vi "initalize dual gating(SubVI).vi"(0 "簇":T1={"initialize"=enum."SR830", "6221"={"6221 Resource"="GPIB0::24::INSTR", "Delta status"=FALSE, "电流"=0.0}, "SR830+6221"={"source"=0, "阻抗"=0.0, "量程入 4"=0, "量程入 3"=0, "量程入 2"=0, "量程入 1"=0, "SR830 2"=FALSE, "SR830 3"=FALSE, "SR830 4"=FALSE, "SR830 1"=FALSE, "VISA 1"="", "VISA 2"="", "VISA 3"="", "VISA 4"="", "Reserve 1"=0, "Reserve 2"=-1, "Reserve 3"=-1, "Reserve 4"=-1, "量程"=enum."量程每次测量会判定"}, "2400"={"2400"=FALSE, "VISA"=""}, "ch"={"ch"=[], "current"=[], "change?"=[], "holding current\nwhen change ch?"=FALSE}, "Instrument"={"335 Resource"="GPIB0::24::INSTR", "Input (0:A)"=0, "Instrument Type"=enum."SVSM", "quantum design"=refnum, "Heater Output (1:1)"=1, "semaphore"=refnum, "TCP master instance"=refnum, "335 Status"=refnum, "M24C Resource"="GPIB0::24::INSTR", "4G supply"="GPIB0::24::INSTR", "Temp Status 24C"=refnum, "Temp"=refnum, "9T信号"=refnum, "limit"={"Field limit"=0.0, "Field rate limit"=0.0, "Temp limit"=0.0, "Temp low limit"=0.0, "Temp rate limit "=0.0}, "4g supply status"=refnum, "vi路径"=""}, "Aborting"=refnum, "数据文件"=refnum, "warning"=refnum, "2614B"={"2614B chA"=FALSE, "2614B chB"=FALSE, "VISA"=""}} {"Instrument"."Input (0:A)" items=["A", "B"]; "Instrument"."Heater Output (1:1)" items=["1"=1, "2"=2]; "SR830+6221"."Reserve 4" items=["Auto Reserve"=-1, "High Reserve"=0, "Normal"=1, "Low Noise"=2]; "SR830+6221"."Reserve 3" items=["Auto Reserve"=-1, "High Reserve"=0, "Normal"=1, "Low Noise"=2]; "SR830+6221"."Reserve 2" items=["Auto Reserve"=-1, "High Reserve"=0, "Normal"=1, "Low Noise"=2]; "SR830+6221"."Reserve 1" items=["量程每次测量会判定", "量程不变为设定值"]; "SR830+6221"."source" items=["SR830 1", "SR830 2", "SR830 3", "SR830 4"]}, 2 "字符串":string) -> (7 "输出簇":T1={"initialize"=enum."SR830", "6221"={"6221 Resource"="GPIB0::24::INSTR", "Delta status"=FALSE, "电流"=0.0}, "SR830+6221"={"source"=0, "阻抗"=0.0, "量程入 4"=0, "量程入 3"=0, "量程入 2"=0, "量程入 1"=0, "SR830 2"=FALSE, "SR830 3"=FALSE, "SR830 4"=FALSE, "SR830 1"=FALSE, "VISA 1"="", "VISA 2"="", "VISA 3"="", "VISA 4"="", "Reserve 1"=0, "Reserve 2"=-1, "Reserve 3"=-1, "Reserve 4"=-1, "量程"=enum."量程每次测量会判定"}, "2400"={"2400"=FALSE, "VISA"=""}, "ch"={"ch"=[], "current"=[], "change?"=[], "holding current\nwhen change ch?"=FALSE}, "Instrument"={"335 Resource"="GPIB0::24::INSTR", "Input (0:A)"=0, "Instrument Type"=enum."SVSM", "quantum design"=refnum, "Heater Output (1:1)"=1, "semaphore"=refnum, "TCP master instance"=refnum, "335 Status"=refnum, "M24C Resource"="GPIB0::24::INSTR", "4G supply"="GPIB0::24::INSTR", "Temp Status 24C"=refnum, "Temp"=refnum, "9T信号"=refnum, "limit"={"Field limit"=0.0, "Field rate limit"=0.0, "Temp limit"=0.0, "Temp low limit"=0.0, "Temp rate limit "=0.0}, "4g supply status"=refnum, "vi路径"=""}, "Aborting"=refnum, "数据文件"=refnum, "warning"=refnum, "2614B"={"2614B chA"=FALSE, "2614B chB"=FALSE, "VISA"=""}} {"Instrument"."Input (0:A)" items=["A", "B"]; "Instrument"."Heater Output (1:1)" items=["1"=1, "2"=2]; "SR830+6221"."Reserve 4" items=["Auto Reserve"=-1, "High Reserve"=0, "Normal"=1, "Low Noise"=2]; "SR830+6221"."Reserve 3" items=["Auto Reserve"=-1, "High Reserve"=0, "Normal"=1, "Low Noise"=2]; "SR830+6221"."Reserve 2" items=["Auto Reserve"=-1, "High Reserve"=0, "Normal"=1, "Low Noise"=2]; "SR830+6221"."Reserve 1" items=["量程每次测量会判定", "量程不变为设定值"]; "SR830+6221"."source" items=["SR830 1", "SR830 2", "SR830 3", "SR830 4"]})   [LabVIEW 2019, in "initialize.lvlib"]
uses:
  initialize.lvlib
  config.ctl
  <vilib>/NI/Modbus Library/API/Master/Modbus Master.lvclass
  initialize.ctl
  Instrument.ctl
  Instrument Type.ctl
  lib/QDInstrument.dll
  335 state.ctl
  limit.ctl
  9T mag field stauts.ctl
  warning.ctl
  lib/Keithley 2600 Series/Public/Configure/Source/Configure Source (Range).vi
  lib/Keithley 2600 Series/Public/Configure/Source/Configure Source (Limit).vi
  lib/Keithley 2600 Series/Keithley 2600 Series.lvlib
panel:
  in  "chB":bool
  in  "chA":bool
  in  "Current Limit B (0.1 A) 2":dbl=0.1
  in  "Current Limit A (0.1 A)":dbl=0.1
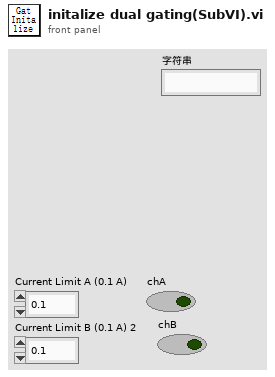
[diagram p1: front panel]
types:
  T1 = typedef "config.ctl" = cluster{"initialize":T2, "6221":cluster{"6221 Resource":refnum<visa-resource-name>, "Delta status":bool, "电流":dbl}, "SR830+6221":cluster{"source":u16, "阻抗":dbl, "量程入 4":i32, "量程入 3":i32, "量程入 2":i32, "量程入 1":i32, "SR830 2":bool, "SR830 3":bool, "SR830 4":bool, "SR830 1":bool, "VISA 1":refnum<visa-resource-name>, "VISA 2":refnum<visa-resource-name>, "VISA 3":refnum<visa-resource-name>, "VISA 4":refnum<visa-resource-name>, "Reserve 1":i16, "Reserve 2":i16, "Reserve 3":i16, "Reserve 4":i16, "量程":enum16{"量程每次测量会判定", "量程不变为设定值"}}, "2400":cluster{"2400":bool, "VISA":refnum<visa-resource-name>}, "ch":cluster{"ch":i32[], "current":dbl[], "change?":bool[], "holding current\nwhen change ch?":bool}, "Instrument":T3, "Aborting":refnum<vi>, "数据文件":refnum<vi>, "warning":refnum<vi>, "2614B":cluster{"2614B chA":bool, "2614B chB":bool, "VISA":refnum<visa-resource-name>}}
  T2 = typedef "initialize.ctl" = enum16{"SR830", "keithley6221-SR830", "Delta", "Delta-tunnelling", "keithley6221-2182-DC"}
  T3 = typedef "Instrument.ctl" = cluster{"335 Resource":refnum<visa-resource-name>, "Input (0:A)":u16, "Instrument Type":T4, "quantum design":refnum<k24>, "Heater Output (1:1)":u16, "semaphore":T5, "TCP master instance":refnum<class "Modbus Master.lvclass">, "335 Status":refnum<vi>, "M24C Resource":refnum<visa-resource-name>, "4G supply":refnum<visa-resource-name>, "Temp Status 24C":refnum<vi>, "Temp":refnum<vi>, "9T信号":T5, "limit":T6, "4g supply status":refnum<vi>, "vi路径":string}
  T4 = typedef "Instrument Type.ctl" = enum16{"PPMS", "VersaLab", "DynaCool", "SVSM", "PPMS-Rotate", "Lakeshore335", "9T mag"}
  T5 = typedef "Semaphore RefNum" = refnum<k1>
  T6 = typedef "limit.ctl" = cluster{"Field limit":dbl, "Field rate limit":dbl, "Temp limit":dbl, "Temp low limit":dbl, "Temp rate limit ":dbl}
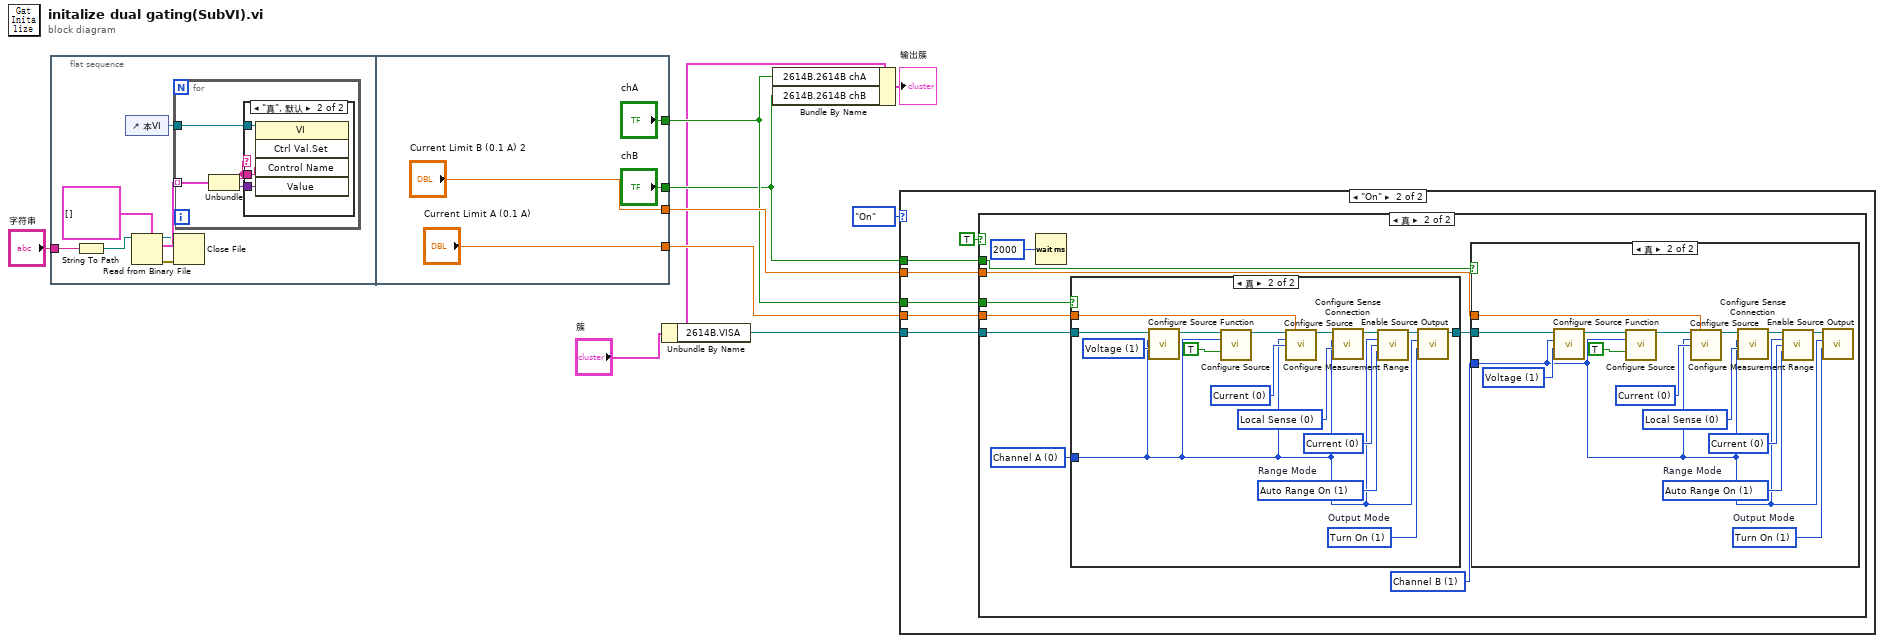
[diagram p0: block diagram]
diagram:
  n1 = flat-sequence {
    tunnel: "字符串" -> [w10]
    tunnel: ["chA"] -> w4
    tunnel: ["Current Limit A (0.1 A)"] -> w5
    tunnel: ["Current Limit B (0.1 A) 2"] -> w6
    tunnel: ["chB"] -> w3
    frame #0 {
      n2 = String To Path(string=w10) -> (path=w15:path)
      n3 = control-ref of="本VI"() -> (w16:refnum<vi>)
      n4 = Read from Binary File(5:cluster{"Name":string, "Variant Data":variant}[] [] ("控件值:获取全部"), 11:w15) -> (0:w11:errorcluster, 2:w13:cluster{"Name":string, "Variant Data":variant}[], 3:w12:refnum<file>)  [unwired: 4 in, 1 out]
      n5 = for {
        tunnel: w13 -> [w20] mode=indexing
        tunnel: w16 -> [w19]
        n6 = Unbundle(w20) -> ("Name"=w17:string, "Variant Data"=w18:variant)
        n7 = case shown="\"真\", 默认" w17 {
          tunnel: w19 -> [_ w23]
          tunnel: w17 -> [_ w22]
          tunnel: w18 -> [_ w21]
          frame "cancel", "load", "model", "ok" {
          }
          frame "真", Default {
            n8 = invoke class="VI" method="Ctrl Val.Set"(reference=w23, "Control Name"=w22, "Value"=w21) -> ()  [unwired: 2 in, 5 out]
          }
        }
      }
      n9 = Close File(refnum=w12, error in=w11) -> ()  [unwired: 2 out]
    }
    frame #1 {
    }
  }
  n10 = Unbundle By Name("簇") -> ("2614B.VISA"=w1:refnum<visa-resource-name>)
  n11 = Bundle By Name(cluster="簇", "2614B.2614B chA"=w4, "2614B.2614B chB"=w3) -> (→"输出簇":T1)
  n12 = case shown="\"On\"" enum16{"Off", "On"}."On" ("Output State") {
    tunnel: w3 -> [_ w32]
    tunnel: w6 -> [_ w31]
    tunnel: w4 -> [_ w30]
    tunnel: w1 -> [_ w29]
    tunnel: w5 -> [_ w28]
    frame "Off", Default {
    }
    frame "On" {
      n13 = case shown="真" TRUE {
        tunnel: w32 -> [_ w40]
        tunnel: w31 -> [_ w38]
        tunnel: w30 -> [_ w37]
        tunnel: w29 -> [_ w36]
        tunnel: w28 -> [_ w34]
        frame False {
        }
        frame True {
          w35 = 0 items=["Channel A", "Channel B"] ("Source Measure Unit Channel (0: Channel A)")
          w39 = 1 items=["Channel A", "Channel B"] ("Source Measure Unit Channel (0: Channel A)")
          n14 = Wait (ms)(milliseconds to wait=u32 2000) -> ()  [unwired: 1 out]
          n15 = case shown="真" w37 {
            tunnel: w36 -> [w58 w64]
            tunnel: w35 -> [_ w63]
            tunnel: w34 -> [_ w61]
            tunnel: [w58 w59] -> w41
            frame False {
            }
            frame True {
              w70 = 0 items=["Local Sense", "Remote Sense"] ("Sense Mode (0: Local Sense)")
              w69 = 0 items=["Current", "Voltage"] ("Range Type (0: Current)")
              w67 = 0 items=["Current", "Voltage", "Power"] ("Limit Type (1: Voltage)")
              w65 = 1 items=["Current", "Voltage"] ("Source Function (1: Voltage)")
              w68 = 1 items=["Auto Range Off", "Auto Range On", "Auto Range Follow Limit"]  # Range Mode
              w71 = 1 items=["Turn off", "Turn On", "High-Z"]  # Output Mode
              n16 = call "Configure Source Function.vi"("Source Function (1: Voltage)"=w65, "Source Measure Unit Channel (0: Channel A)"=w63, "VISA resource name"=w64) -> ("VISA resource name out"=w72:refnum<visa-resource-name>)  [unwired: 7 in, 1 out]
              n17 = call-poly "Configure Source.vi"("VISA resource name"=w72, "Source Measure Unit Channel (0: Channel A)"=w63, "Auto Range (T: Enable)"=TRUE) -> ("VISA resource name out"=w73:refnum<visa-resource-name>)  [unwired: 11 in, 1 out]
              n18 = call-poly "Configure Source.vi"("VISA resource name"=w73, "Current Limit (0.1 A)"=w61, "Source Measure Unit Channel (0: Channel A)"=w63, "Limit Type (1: Voltage)"=w67) -> ("VISA resource name out"=w74:refnum<visa-resource-name>)  [unwired: 10 in, 1 out]
              n19 = call "Configure Sense Connection.vi"("Sense Mode (0: Local Sense)"=w70, "Source Measure Unit Channel (0: Channel A)"=w63, "VISA resource name"=w74) -> ("VISA resource name out"=w62:refnum<visa-resource-name>)  [unwired: 7 in, 1 out]
              n20 = call "Configure Measurement Range.vi"("VISA resource name"=w62, "Source Measure Unit Channel (0: Channel A)"=w63, "Range Type (0: Current)"=w69, "Range Mode (1: Auto Range On)"=w68) -> ("VISA resource name out"=w60:refnum<visa-resource-name>)  [unwired: 10 in, 1 out]
              n21 = call "Enable Source Output.vi"("Output Mode (0: Turn off)"=w71, "Source Measure Unit Channel (0: Channel A)"=w63, "VISA resource name"=w60) -> ("VISA resource name out"=w59:refnum<visa-resource-name>)  [unwired: 7 in, 1 out]
            }
          }
          n22 = case shown="真" w40 {
            tunnel: w41 -> [_ w47]
            tunnel: w39 -> [_ w46]
            tunnel: w38 -> [_ w44]
            frame False {
            }
            frame True {
              w53 = 0 items=["Local Sense", "Remote Sense"] ("Sense Mode (0: Local Sense)")
              w52 = 0 items=["Current", "Voltage"] ("Range Type (0: Current)")
              w50 = 0 items=["Current", "Voltage", "Power"] ("Limit Type (1: Voltage)")
              w48 = 1 items=["Current", "Voltage"] ("Source Function (1: Voltage)")
              w51 = 1 items=["Auto Range Off", "Auto Range On", "Auto Range Follow Limit"]  # Range Mode
              w54 = 1 items=["Turn off", "Turn On", "High-Z"]  # Output Mode
              n23 = call "Configure Source Function.vi"("Source Function (1: Voltage)"=w48, "Source Measure Unit Channel (0: Channel A)"=w46, "VISA resource name"=w47) -> ("VISA resource name out"=w55:refnum<visa-resource-name>)  [unwired: 7 in, 1 out]
              n24 = call-poly "Configure Source.vi"("VISA resource name"=w55, "Source Measure Unit Channel (0: Channel A)"=w46, "Auto Range (T: Enable)"=TRUE) -> ("VISA resource name out"=w56:refnum<visa-resource-name>)  [unwired: 11 in, 1 out]
              n25 = call-poly "Configure Source.vi"("VISA resource name"=w56, "Current Limit (0.1 A)"=w44, "Source Measure Unit Channel (0: Channel A)"=w46, "Limit Type (1: Voltage)"=w50) -> ("VISA resource name out"=w57:refnum<visa-resource-name>)  [unwired: 10 in, 1 out]
              n26 = call "Configure Sense Connection.vi"("Sense Mode (0: Local Sense)"=w53, "Source Measure Unit Channel (0: Channel A)"=w46, "VISA resource name"=w57) -> ("VISA resource name out"=w45:refnum<visa-resource-name>)  [unwired: 7 in, 1 out]
              n27 = call "Configure Measurement Range.vi"("VISA resource name"=w45, "Source Measure Unit Channel (0: Channel A)"=w46, "Range Type (0: Current)"=w52, "Range Mode (1: Auto Range On)"=w51) -> ("VISA resource name out"=w43:refnum<visa-resource-name>)  [unwired: 10 in, 1 out]
              n28 = call "Enable Source Output.vi"("Output Mode (0: Turn off)"=w54, "Source Measure Unit Channel (0: Channel A)"=w46, "VISA resource name"=w43) -> ()  [unwired: 7 in, 2 out]
            }
          }
        }
      }
    }
  }
